vi "action_define_spectrum.vi"(2 "action data":T1[](array[typedef]) {"par 4" format="%.2f"; "par 3" format="%.2f"; "par 2" format="%.2f"; "par" format="%.2f"}, 5 "error in (no error)":errorcluster) -> (16 "action data out":T1[](array[typedef]) {"par 4" format="%.2f"; "par 3" format="%.2f"; "par 2" format="%.2f"; "par" format="%.2f"}, 19 "error out":errorcluster)   [LabVIEW 2010, in "OSA.lvclass"]
doc: "SubVI to a <B>Thorlabs_OSA_64</B> object.\n\n[GOOP 1.0]"
uses:
  OSA.lvclass
  action_data.ctl
  typeDef/queue_action.ctl
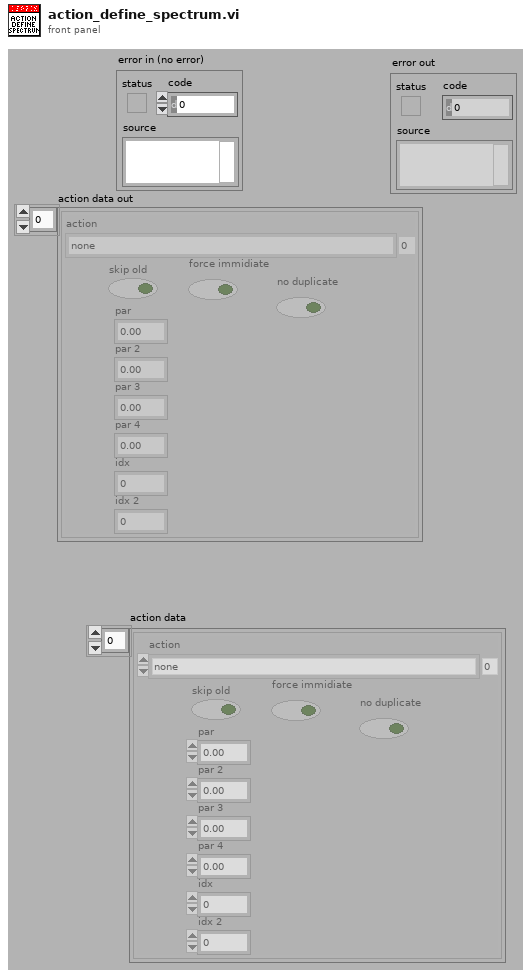
[diagram p1: front panel]
types:
  T1 = typedef "OSA.lvclass/action_data.ctl" = cluster{"action":T2, "skip old":bool, "force immidiate":bool, "par":dbl, "par 2":dbl, "par 3":dbl, "par 4":dbl, "idx":i32, "idx 2":i32, "no duplicate":bool}
  T2 = typedef "OSA.lvclass/queue_action.ctl" = enum16{"none", "stop", "GUI_plotInterferogram", "GUI_plotSpectrum", "GUI_plotInterferogramRescale", "GUI_plotSpectrumRescale", "GUI_plotInterferogramReset", "GUI_plotSpectrumReset", "GUI_plotInterferogramAutoScaleY", "GUI_plotSpectrumAutoScaleY", "GUI_plotInterferogramZoomOut", "GUI_plotSpectrumZoomOut", "GUI_plotInterferogramPane", "GUI_plotSpectrumPane", "GUI_plotInterferogramZoomMouse", "GUI_plotSpectrumZoomMouse", "GUI_spectrumChannelType", "GUI_channel", "ENVIRONMENT temperature", "ENVIRONMENT pressure", "MODE_resolution set", "MODE_resolution get", "MODE_sensitivity set", "MODE_sensitivity get", "MODE_PDTemperature set", "MODE_PDTemperature get", "REBOOT/RESET firmware", "ACQASYNC_acquireSingleSpectrum", "ACQASYNC_continuous start", "ACQASYNC_continuous stop\n", "ACQASYNC_get last interferogram", "ACQASYNC_get last spectrum", "ACQASYNC_get last waveNr", "ACQOPT_interferogram smoothing set", "ACQOPT_interferogram smoothing get", "ACQOPT_spectrum smoothing set", "ACQOPT_spectrum smoothing get", "ACQOPT_apodisation type set", "ACQOPT_apodisation type get", "ACQOPT_phase correction type set", "ACQOPT_phase correction type get", "ACQOPT_acqIntervall_set", "ACQOPT_acqIntervall_get", "ACQOPT_average spectrum set", "ACQOPT_average spectrum get", "ACQOPT_rolling average set", "ACQOPT_rolling average get", "ACQOPT_zero fill factor set", "ACQOPT_zero fill factor get", "ACQOPT_cycle counting set", "ACQOPT_cycle counting get", "ACQOPT_air measure option set", "ACQOPT_air measure option get", "ACQOPT_gainLevel auto get", "ACQOPT_gainLevel auto set", "ACQOPT_gainLevel get", "ACQOPT_gainLevel set", "ACQOPT_getAll", "INSTRUMENT_PROPERTY_range_WaveNr_min", "INSTRUMENT_PROPERTY_range_WaveNr_max", "INSTRUMENT_PROPERTY_reference_wavelength_cm^-1", "INSTRUMENT_PROPERTY_samplesPerRefPeriod", "INSTRUMENT_PROPERTY_resolution_waveNrPercm", "INSTRUMENT_PROPERTY_availableGainLevels", "INSTRUMENT_PROPERTY_status", "CONVERT", "ANALYSE_POWER", "ANALYSE_PEAKS", "ANALYSE_WAVELENGTH", "ANALYSE_SPECTRUM", "ANALYSE_INTERFEROGRAM", "ANALYSE_COHERENCE_LENGTH", "MATH", "MATH_power", "MATH_peaks", "FILE", "miscellaneous"}
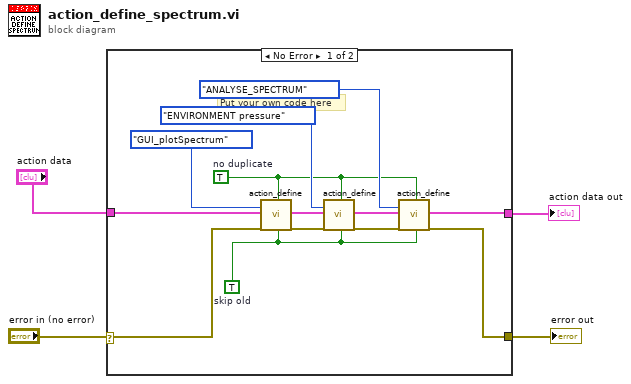
[diagram p0: block diagram]
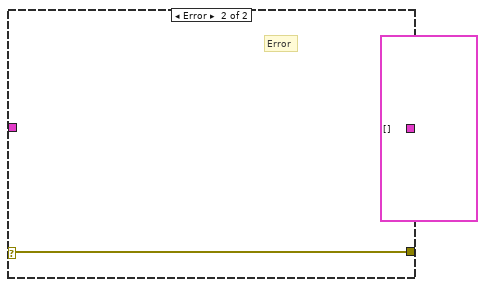
[diagram p2: hidden frame]
diagram:
  n1 = case shown="No Error" "error in (no error)" {
    selector: "error in (no error)" -> [w12 w19]
    tunnel: [w11 w19] -> w4
    tunnel: [w10 T1[] [] ("action data out")] -> w2
    tunnel: "action data" -> [w9 _]
    frame No Error {
      w5 = TRUE  # no duplicate
      w8 = TRUE  # skip old
      # "Put your own code here"
      n2 = call "action_define.vi"("action"=queue_action."GUI_plotSpectrum", "action data"=w9, "error in (no error)"=w12, "no duplicate"=w5, "skip old"=w8) -> ("action data out"=w16:T1[], "error out"=w17:errorcluster)  [unwired: 13 in]
      n3 = call "action_define.vi"("action"=queue_action."ENVIRONMENT pressure", "action data"=w16, "error in (no error)"=w17, "no duplicate"=w5, "skip old"=w8) -> ("action data out"=w7:T1[], "error out"=w6:errorcluster)  [unwired: 13 in]
      n4 = call "action_define.vi"("action"=queue_action."ANALYSE_SPECTRUM", "action data"=w7, "error in (no error)"=w6, "no duplicate"=w5, "skip old"=w8) -> ("action data out"=w10:T1[], "error out"=w11:errorcluster)  [unwired: 13 in]
    }
    frame Error {
      # "Error"
    }
  }
  "error out" <- w4
  "action data out" <- w2
